vi "Get Default Sample Period.vi"(4 "error in (no error)":errorcluster, 7 "Plugin Name":T1) -> (0 "error out":errorcluster, 3 "Sample Period (msec)":i32)   [LabVIEW 2015, in "Config Data.lvlib" / "Config Data.lvclass"]
uses:
  Config Data.lvclass
  Startup Processes/_typedefs/Subpanel Names.ctl
  Startup Processes/Startup Processes.lvlib
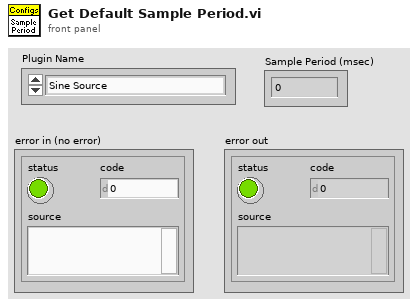
[diagram p1: front panel]
types:
  T1 = typedef "Startup Processes.lvlib/Subpanel Names.ctl" = enum16{"Sine Source", "Ramp Source", "Hen House TC", "Dog House TC", "Out House TC"}
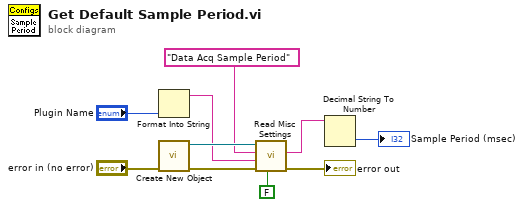
[diagram p0: block diagram]
diagram:
  n1 = Format Into String("Plugin Name") -> (resulting string=w3:string)  [unwired: 3 in, 1 out]
  n2 = call "Create New Object.vi"("Error In"="error in (no error)") -> ("Error Out"=w9:errorcluster, "Config Data"=w10:refnum<class "Config Data.lvclass">)  [unwired: 5 in]
  n3 = call-dynamic "Read Misc Settings.vi"("Reload"=FALSE, "error in (no error)"=w9, "Key"=w3, "Section"="Data Acq Sample Period" ("format string"), "Config Data in"=w10) -> ("error out"=→"error out":errorcluster, "p_value"=w6:string)  [unwired: 1 in, 1 out]
  n4 = Decimal String To Number(string=w6) -> (number=→"Sample Period (msec)":i32)  [unwired: 2 in, 1 out]
